vi "Enqueue for Receive.vi"(6 "priority":i32, 8 "error in (no error)":errorcluster, 9 "timeout ms (-1)":i32=-1, 10 "Message":refnum<class "Message.lvclass">, 11 "AF Queue Stream in":refnum<class "AF Queue Stream.lvclass">) -> (0 "error out":errorcluster, 3 "AF Queue Stream out":refnum<class "AF Queue Stream.lvclass">)   [LabVIEW 2020, in "AF Queue Stream.lvclass"]
doc: "Override this method to specify the action the local copy of this object will perform to send a message to its remote counterpart."
uses:
  AF Queue Stream.lvclass
  <vilib>/ActorFramework/Message Enqueuer/Message Enqueuer.lvclass
  <vilib>/ActorFramework/Message Queue/Message Queue.lvclass
  <vilib>/ActorFramework/Message/Message.lvclass
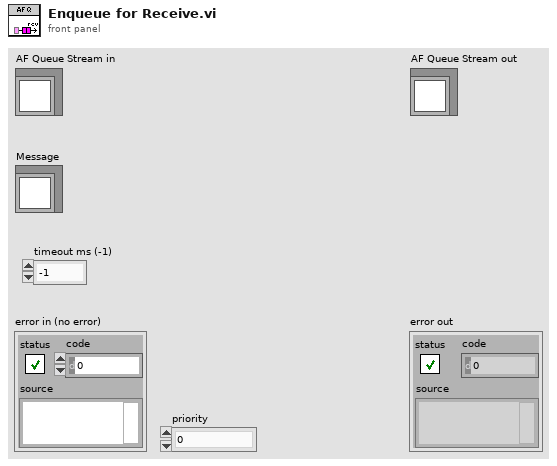
[diagram p1: front panel]
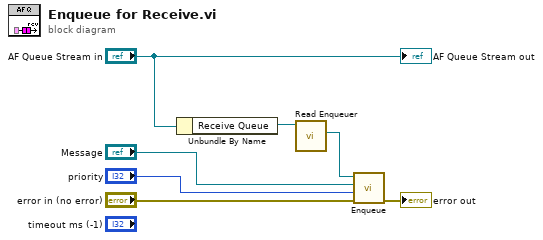
[diagram p0: block diagram]
diagram:
  n1 = Unbundle By Name("AF Queue Stream in") -> ("Receive Queue"=w2:refnum<class "Message Queue.lvclass">)
  n2 = call <vilib>:"Read Enqueuer.vi"("Message Queue"=w2) -> ("Message Enqueuer"=w1:refnum<class "Message Enqueuer.lvclass">)  [unwired: 10 in]
  n3 = call <vilib>:"Enqueue.vi"("error in (no error)"="error in (no error)", "Message Priority (Normal)"="priority", "Message"="Message", "Message Enqueuer in"=w1) -> ("error out"=→"error out":errorcluster)  [unwired: 6 in, 1 out]
  "AF Queue Stream out" <- "AF Queue Stream in"
